vi "bh3_bluetooth_read.vi"(7 "command_expected(x00)":u8 format="%02x", 8 "error in (no error)":errorcluster, 11 "bt connection ID in":refnum<k31>) -> (0 "error out":errorcluster, 2 "response byte array":u8[](array[numeric]), 3 "bt connection ID out":refnum<k31>)   [LabVIEW 2013]
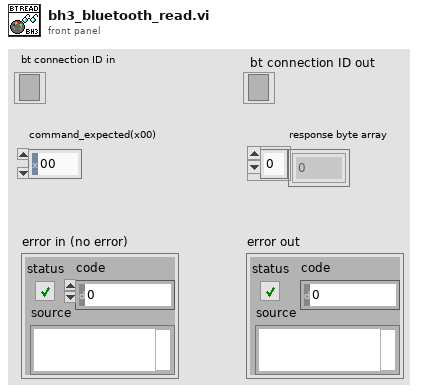
[diagram p1: front panel]
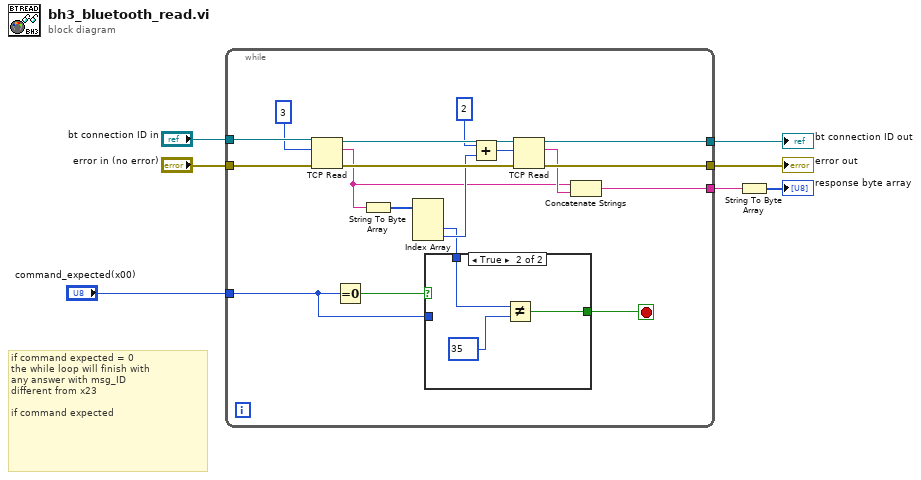
[diagram p0: block diagram]
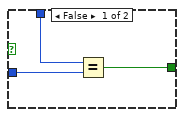
[diagram p2: hidden frame]
diagram:
  # "if command expected = 0\nthe while loop will finish with\nany answer with msg_ID \ndifferent from x23\n\nif command expected"
  n1 = while {
    tunnel: "bt connection ID in" -> [w25]
    tunnel: [w16] -> w6
    tunnel: "error in (no error)" -> [w24]
    tunnel: [w15] -> w4
    tunnel: [w12] -> w2
    tunnel: "command_expected(x00)" -> [w8]
    stop <- w10 stop-if-true
    n2 = TCP Read(connection ID=w25, bytes to read=3, error in (no error)=w24) -> (connection ID out=w21:refnum<k31>, data out=w13:string, error out=w20:errorcluster)  [unwired: 2 in]
    n3 = Equal To 0?(x=w8) -> (x = 0?=w11:bool)
    n4 = String To Byte Array(string=w13) -> (unsigned byte array=w22:u8[])
    n5 = Index Array(array=w22) -> (element #2=w9:u8, element #3=w18:u8)  [unwired: 3 in, 1 out]
    n6 = case shown="True" w11 {
      tunnel: [w28 w31] -> w10
      tunnel: w9 -> [w27 w29]
      tunnel: w8 -> [w26 _]
      frame False {
        n7 = Equal?(x=w27, y=w26) -> (x = y?=w28:bool)
      }
      frame True {
        n8 = Not Equal?(x=w29, y=u8 35 ("bytes to read")) -> (x != y?=w31:bool)
      }
    }
    n9 = Add(x=u8 2, y=w18) -> (x+y=w19:u8)
    n10 = TCP Read(connection ID=w21, bytes to read=w19, error in (no error)=w20) -> (connection ID out=w16:refnum<k31>, data out=w14:string, error out=w15:errorcluster)  [unwired: 2 in]
    n11 = Concatenate Strings(w13, w14) -> (w12:string)
  }
  "bt connection ID out" <- w6
  "error out" <- w4
  n12 = String To Byte Array(string=w2) -> (unsigned byte array=→"response byte array":u8[])
